vi "Controller Monitoring Loop.vi"(7 "Sync Objects":T1, 8 "error in (no error)":errorcluster, 11 "FOFB Configuration":T4={"FOFB Parameters"={"Network"={"FOFB Controller IP"="", "LNLS Control Network IP"="", "LNLS Control Network Power Supplies TCP Port"=0, "LNLS Control Network FOFB Configuration TCP Port"=0, "LNLS Control Network BPMs TCP Port"=0, "Monitoring Data TCP Port"=0, "Fast Archiver TCP Port"=0, "Fast Command TCP Port"=0, "TCP Listening Timeout"=0}, "Fast Acquisition"={"Sampling Period"=0, "Data Buffer Size"=0, "Monitoring Period"=0}, "Acquisition Network"=[], "Actuation Network"=[]}, "Number of Acquisition Chassis"=0, "Number of Actuation Chassis"=0, "Number of BPM Readings"=0, "BPM Reading Names"=[], "Selected BPM Readings"=[0, 1, 2, 3, 4, 5, 6, 7, 8, 9, 10, 11, 12, 13, 14, 15, 16, 17, 18, 19, 20, 21, 22, 23, 24, 25, 26, 27, 28, 29, 30, 31, 32, 33, 34, 35, 36, 37, 38, 39, 40, 41, 42, 43, 44, 45, 46, 47, 48, 49], "Number of Correctors"=0, "Corrector Names"=[], "Selected Correctors"=[0, 1, 2, 3, 4, 5, 6, 7, 8, 9, 10, 11, 12, 13, 14, 15, 16, 17, 18, 19, 20, 21, 22, 23, 24, 25, 26, 27, 28, 29, 30, 31, 32, 33, 34, 35, 36, 37, 38, 39, 40, 41, 42, 43, 44, 45, 46, 47, 48, 49], "Response Matrix"=[], "Reference Orbit"=[], "Correction Matrix"=[], "FPGA Filter Sets"=[], "Acquisition Chassis Names"=[], "Actuation Chassis Names"=[], "Acquisition Variables"=[], "Actuation Variables"=[], "PS Matrix Mapping"=[], "Inverse PS Matrix Mapping"=[], "BPM Matrix Mapping"=[], "Inverse BPM Matrix Mapping"=[], "BPM Planes"=[], "Corrector Planes"=[]}) -> (0 "error out":errorcluster)   [LabVIEW 2011, in "Controller VIs.lvlib"]
uses:
  Controller VIs.lvlib
  Types Definitions/Type FOFB Configuration.ctl
  Types Definitions/Type FOFB Parameters.ctl
  Types Definitions/Type Network Configuration.ctl
  Types Definitions/Type FA Configuration.ctl
  Types Definitions/Type Acquisition Network Configuration.ctl
  Types Definitions/Type Actuation Network Configuration.ctl
  Types Definitions/Type Synchronization Objects.ctl
  Types Definitions/Type Blocking Synchronization Objects.ctl
  Types Definitions/Type Monitoring Data.ctl
  Types Definitions/Type Operation Mode State.ctl
  Types Definitions/Type Diagnostics Data.ctl
  Types Definitions/Type CPU Loads Array.ctl
  Types Definitions/Type CPU Loads.ctl
  Types Definitions/Type Non-blocking Synchronization Objects.ctl
  Types Definitions/Type FOFB Variables.ctl
  Types Definitions/Type Actuation State.ctl
  Types Definitions/Type TCP State.ctl
  <vilib>/Platform/TimedLoop/XDataNode/timing_clust.ctl
  <vilib>/Platform/TimedLoop/XDataNode/nitl_modes.ctl
  <vilib>/Platform/TimedLoop/XDataNode/wakeup.ctl
  Controller Global Variables/LNLS Control FOFB Configuration Out.vi
  Controller Global Variables/Monitoring Data.vi
  <vilib>/Platform/TimedLoop/XDataNode/XDataNode.xnode
  Type Definitions.lvlib
  <vilib>/NI_Real-Time Target Support.lvlib
  Controller Global Variables.lvlib
  <vilib>/Platform/TimedLoop/XDataNode/XDNodeRunTimeDep.lvlib
  Filter VIs.lvlib
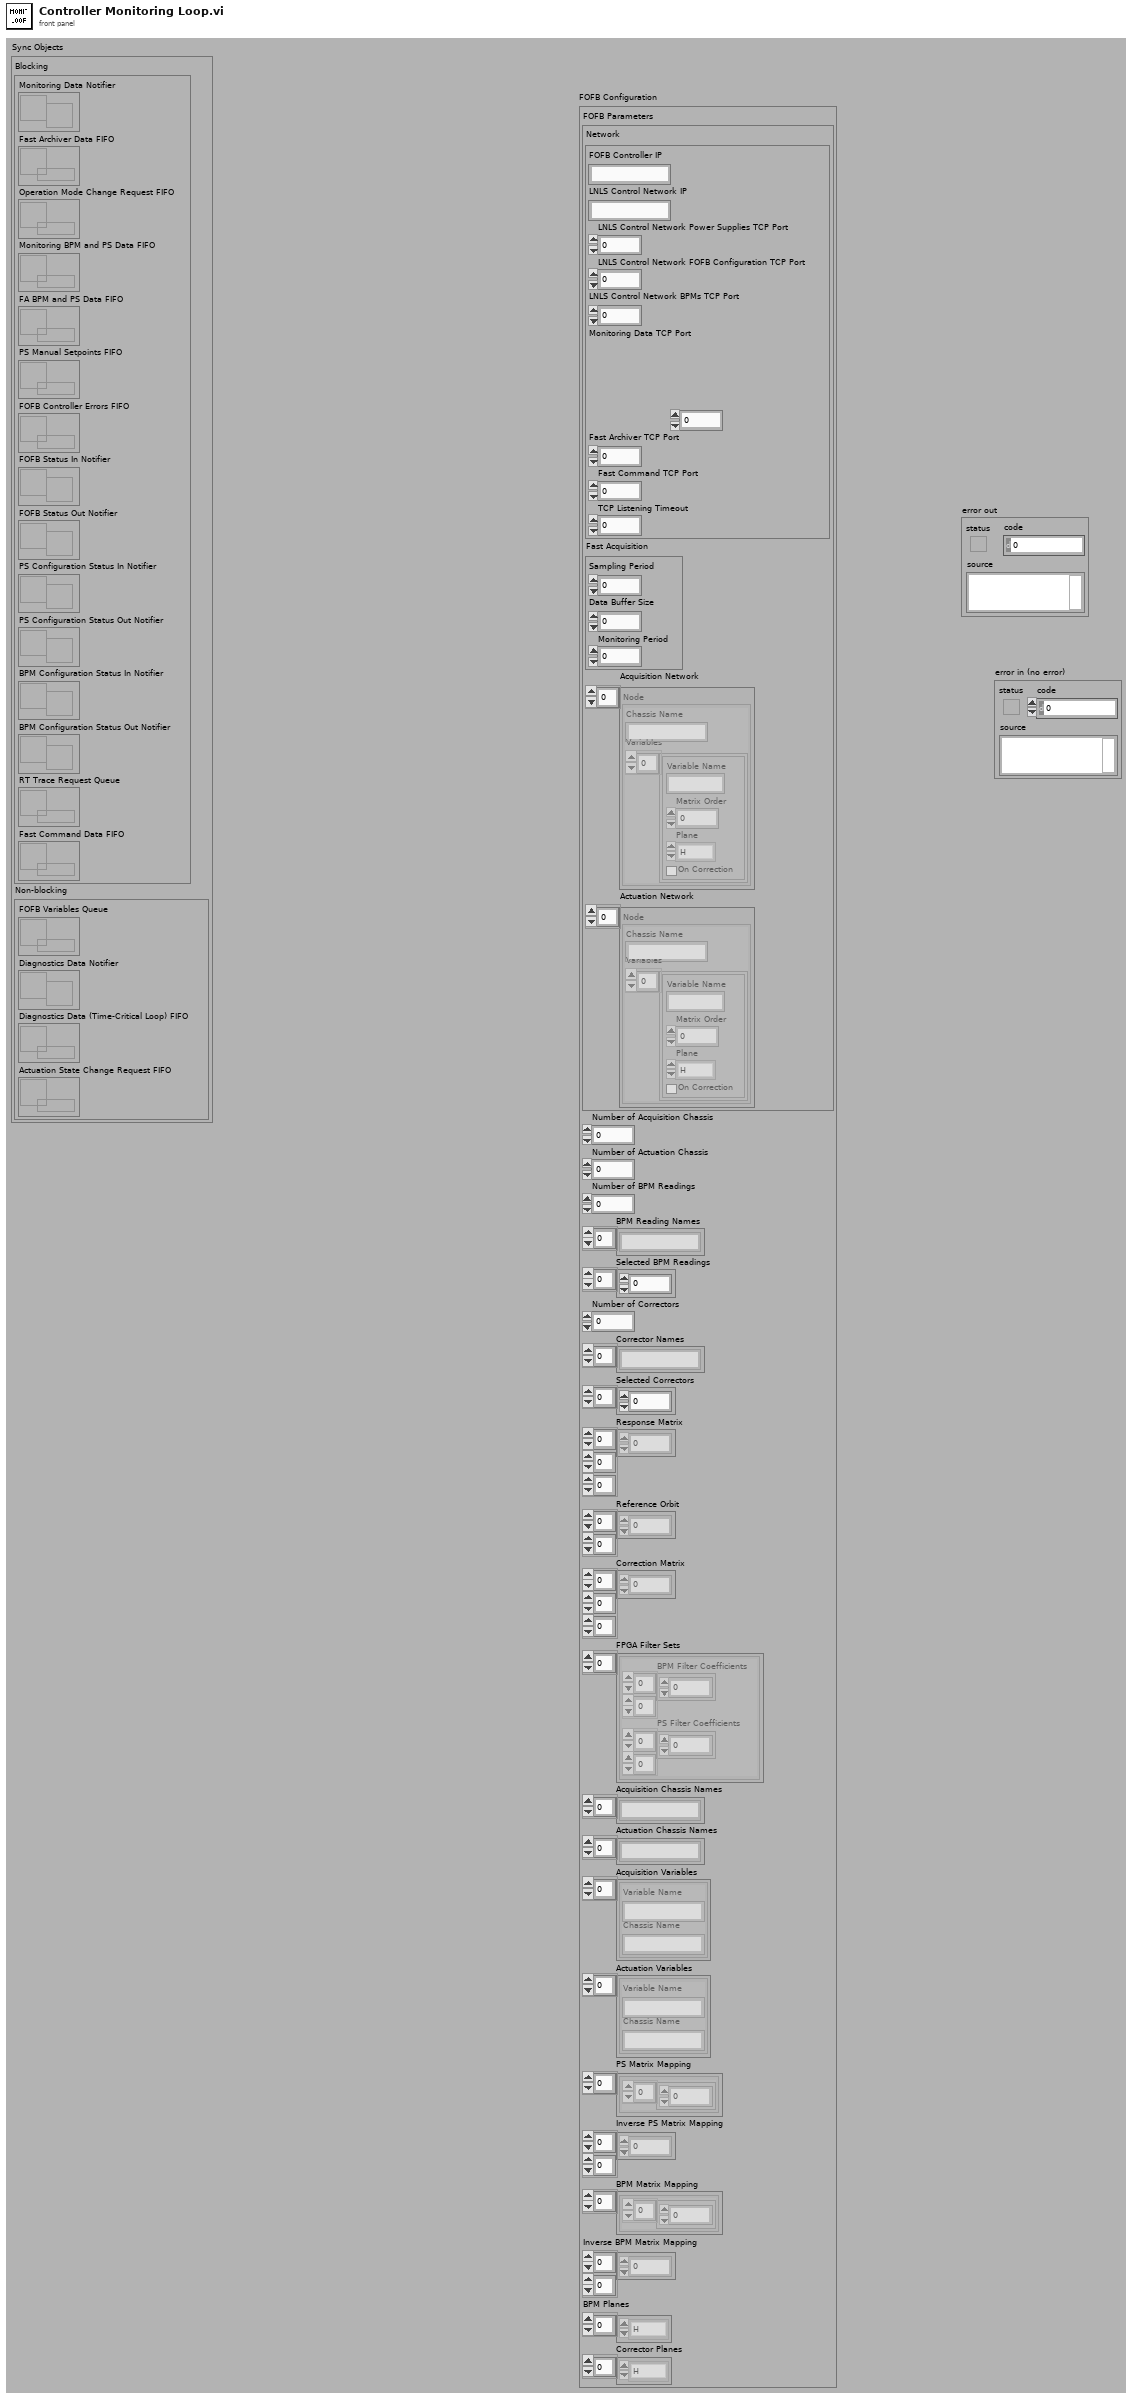
[diagram p1: front panel]
types:
  T1 = typedef "Type Definitions.lvlib/Type Synchronization Objects.ctl" = cluster{"Blocking":T2, "Non-blocking":T3}
  T2 = typedef "Type Definitions.lvlib/Type Blocking Synchronization Objects.ctl" = cluster{"Monitoring Data Notifier":refnum<notifier>, "Fast Archiver Data FIFO":refnum<queue>, "Operation Mode Change Request FIFO":refnum<k33>, "Monitoring BPM and PS Data FIFO":refnum<k33>, "FA BPM and PS Data FIFO":refnum<k33>, "PS Manual Setpoints FIFO":refnum<k33>, "FOFB Controller Errors FIFO ":refnum<k33>, "FOFB Status In Notifier":refnum<notifier>, "FOFB Status Out Notifier":refnum<notifier>, "PS Configuration Status In Notifier":refnum<notifier>, "PS Configuration Status Out Notifier":refnum<notifier>, "BPM Configuration Status In Notifier":refnum<notifier>, "BPM Configuration Status Out Notifier":refnum<notifier>, "RT Trace Request Queue":refnum<queue>, "Fast Command Data FIFO":refnum<k33>}
  T3 = typedef "Type Definitions.lvlib/Type Non-blocking Synchronization Objects.ctl" = cluster{"FOFB Variables Queue":refnum<queue>, "Diagnostics Data Notifier":refnum<notifier>, "Diagnostics Data (Time-Critical Loop) FIFO":refnum<k33>, "Actuation State Change Request FIFO":refnum<k33>}
  T4 = typedef "Type Definitions.lvlib/Type FOFB Configuration.ctl" = cluster{"FOFB Parameters":T5, "Number of Acquisition Chassis":i32, "Number of Actuation Chassis":i32, "Number of BPM Readings":i32, "BPM Reading Names":string[], "Selected BPM Readings":u32[], "Number of Correctors":i32, "Corrector Names":string[], "Selected Correctors":u32[], "Response Matrix":dbl[][][], "Reference Orbit":dbl[][], "Correction Matrix":dbl[][][], "FPGA Filter Sets":cluster{"BPM Filter Coefficients":dbl[][], "PS Filter Coefficients":dbl[][]}[], "Acquisition Chassis Names":string[], "Actuation Chassis Names":string[], "Acquisition Variables":cluster{"Variable Name":string, "Chassis Name":string}[], "Actuation Variables":cluster{"Variable Name":string, "Chassis Name":string}[], "PS Matrix Mapping":cluster{u32[]}[], "Inverse PS Matrix Mapping":u32[][], "BPM Matrix Mapping":cluster{u32[]}[], "Inverse BPM Matrix Mapping":u32[][], "BPM Planes":enum8{"H", "V"}[], "Corrector Planes":enum8{"H", "V"}[]}
  T5 = typedef "Type Definitions.lvlib/Type FOFB Parameters.ctl" = cluster{"Network":T6, "Fast Acquisition":T7, "Acquisition Network":T8, "Actuation Network":T9}
  T6 = typedef "Type Definitions.lvlib/Type Network Configuration.ctl" = cluster{"FOFB Controller IP":string, "LNLS Control Network IP":string, "LNLS Control Network Power Supplies TCP Port":u16, "LNLS Control Network FOFB Configuration TCP Port":u16, "LNLS Control Network BPMs TCP Port":u16, "Monitoring Data TCP Port":u16, "Fast Archiver TCP Port":u16, "Fast Command TCP Port":u16, "TCP Listening Timeout":i32}
  T7 = typedef "Type Definitions.lvlib/Type FA Configuration.ctl" = cluster{"Sampling Period":u32, "Data Buffer Size":u32, "Monitoring Period":u32}
  T8 = typedef "Type Definitions.lvlib/Type Acquisition Network Configuration.ctl" = cluster{"Chassis Name":string, "Variables":cluster{"Variable Name":string, "Matrix Order":u32, "Plane":enum8{"H", "V"}, "On Correction":bool}[]}[]
  T9 = typedef "Type Definitions.lvlib/Type Actuation Network Configuration.ctl" = cluster{"Chassis Name":string, "Variables":cluster{"Variable Name":string, "Matrix Order":u32, "Plane":enum8{"H", "V"}, "On Correction":bool}[]}[]
  T10 = typedef "Type Definitions.lvlib/Type TCP State.ctl" = enum16{"Idle", "Wait Connection", "Read Data", "Process Data", "Write Data", "Close Connection"}
  T11 = typedef "XDNodeRunTimeDep.lvlib/timing_clust.ctl" = cluster{"Expected End [f-1]":u64, "Actual End [f-1]":u64, "Finished Late? [f-1]":bool, "Expected End [i-1]":u64, "Actual End [i-1]":u64, "Finished Late? [i-1]":bool, "Expected Start [i]":u64, "Actual Start [i]":u64, "Expected Start [f]":u64, "Actual Start [f]":u64, "Source Name":string, "Structure Name":string, "Period":i64, "Deadline":i64, "Offset":i64, "Start":i64, "Priority":i32, "Timeout":i32, "Mode":T12, "Wakeup Reason":T13, "Error":errorcluster, "Source Type":string, "Secondary Source Type":string, "Global End Time":u64, "Global Start Time":u64, "Frame Duration":u64, "Iteration Duration":u64, "Assigned CPU":i32, "I/O Scan Engine Mode":u32}
  T12 = typedef "XDNodeRunTimeDep.lvlib/nitl_modes.ctl" = enum32{"No Change", "Process missed periods, maintain original phase", "Discard missed periods, maintain original phase", "Process missed periods, ignore original phase", "Discard missed periods, ignore original phase"}
  T13 = typedef "XDNodeRunTimeDep.lvlib/wakeup.ctl" = enum32{"Normal", "Aborted", "Asynchronous wakeup", "Timing source error", "Timed loop error", "Timeout"}
  T14 = typedef "Type Definitions.lvlib/Type Monitoring Data.ctl" = cluster{"Timestamp":timestamp, "BPM Readings":dbl[], "PS Readings":dbl[], "PS FOFB Setpoints":dbl[], "PS Status per Rack":u8[], "PS ON-OFF per Rack":u8[], "Operation Mode":T15, "Diagnostics Data":T16, "Controller Status Table":i32[]}
  T15 = typedef "Type Definitions.lvlib/Type Operation Mode State.ctl" = enum8{"Idle Mode", "Manual Mode", "FOFB Mode"}
  T16 = typedef "Type Definitions.lvlib/Type Diagnostics Data.ctl" = cluster{"Time-Critical Loop Missed Iterations":u32, "Time-Critical Loop Execution Time (usec)":u32, "Available Memory (bytes)":u32, "CPU Loads Array":T17}
  T17 = typedef "Type Definitions.lvlib/Type CPU Loads Array.ctl" = T18[]
  T18 = typedef "Type Definitions.lvlib/Type CPU Loads.ctl" = cluster{"Total (%)":dbl, "Time Critical (%)":dbl, "Timed Structures (%)":dbl, "High (%)":dbl, "Above Normal (%)":dbl, "Normal (%)":dbl, "Background (%)":dbl, "Idle (%)":dbl, "ISR (%)":dbl}
  T19 = typedef "Type Definitions.lvlib/Type Control FOFB Configuration Out.ctl" = cluster{"Status":u16, "Operation Mode":T15, "Horizontal Gain":sgl, "Vertical Gain":sgl, "Selected Reference Orbit":i32, "Selected Correction Matrix":i32, "Selected FPGA Filters":i32, "Horizontal Distortion Threshold":sgl, "Vertical Distortion Threshold":sgl, "Timestamp":dbl}
  T20 = typedef "NI_Real-Time Target Support.lvlib/RT CPU Load.ctl" = cluster{"Total (%)":dbl, "Time Critical (%)":dbl, "Timed Structures (%)":dbl, "High (%)":dbl, "Above Normal (%)":dbl, "Normal (%)":dbl, "Background (%)":dbl, "Idle (%)":dbl, "ISR (%)":dbl}
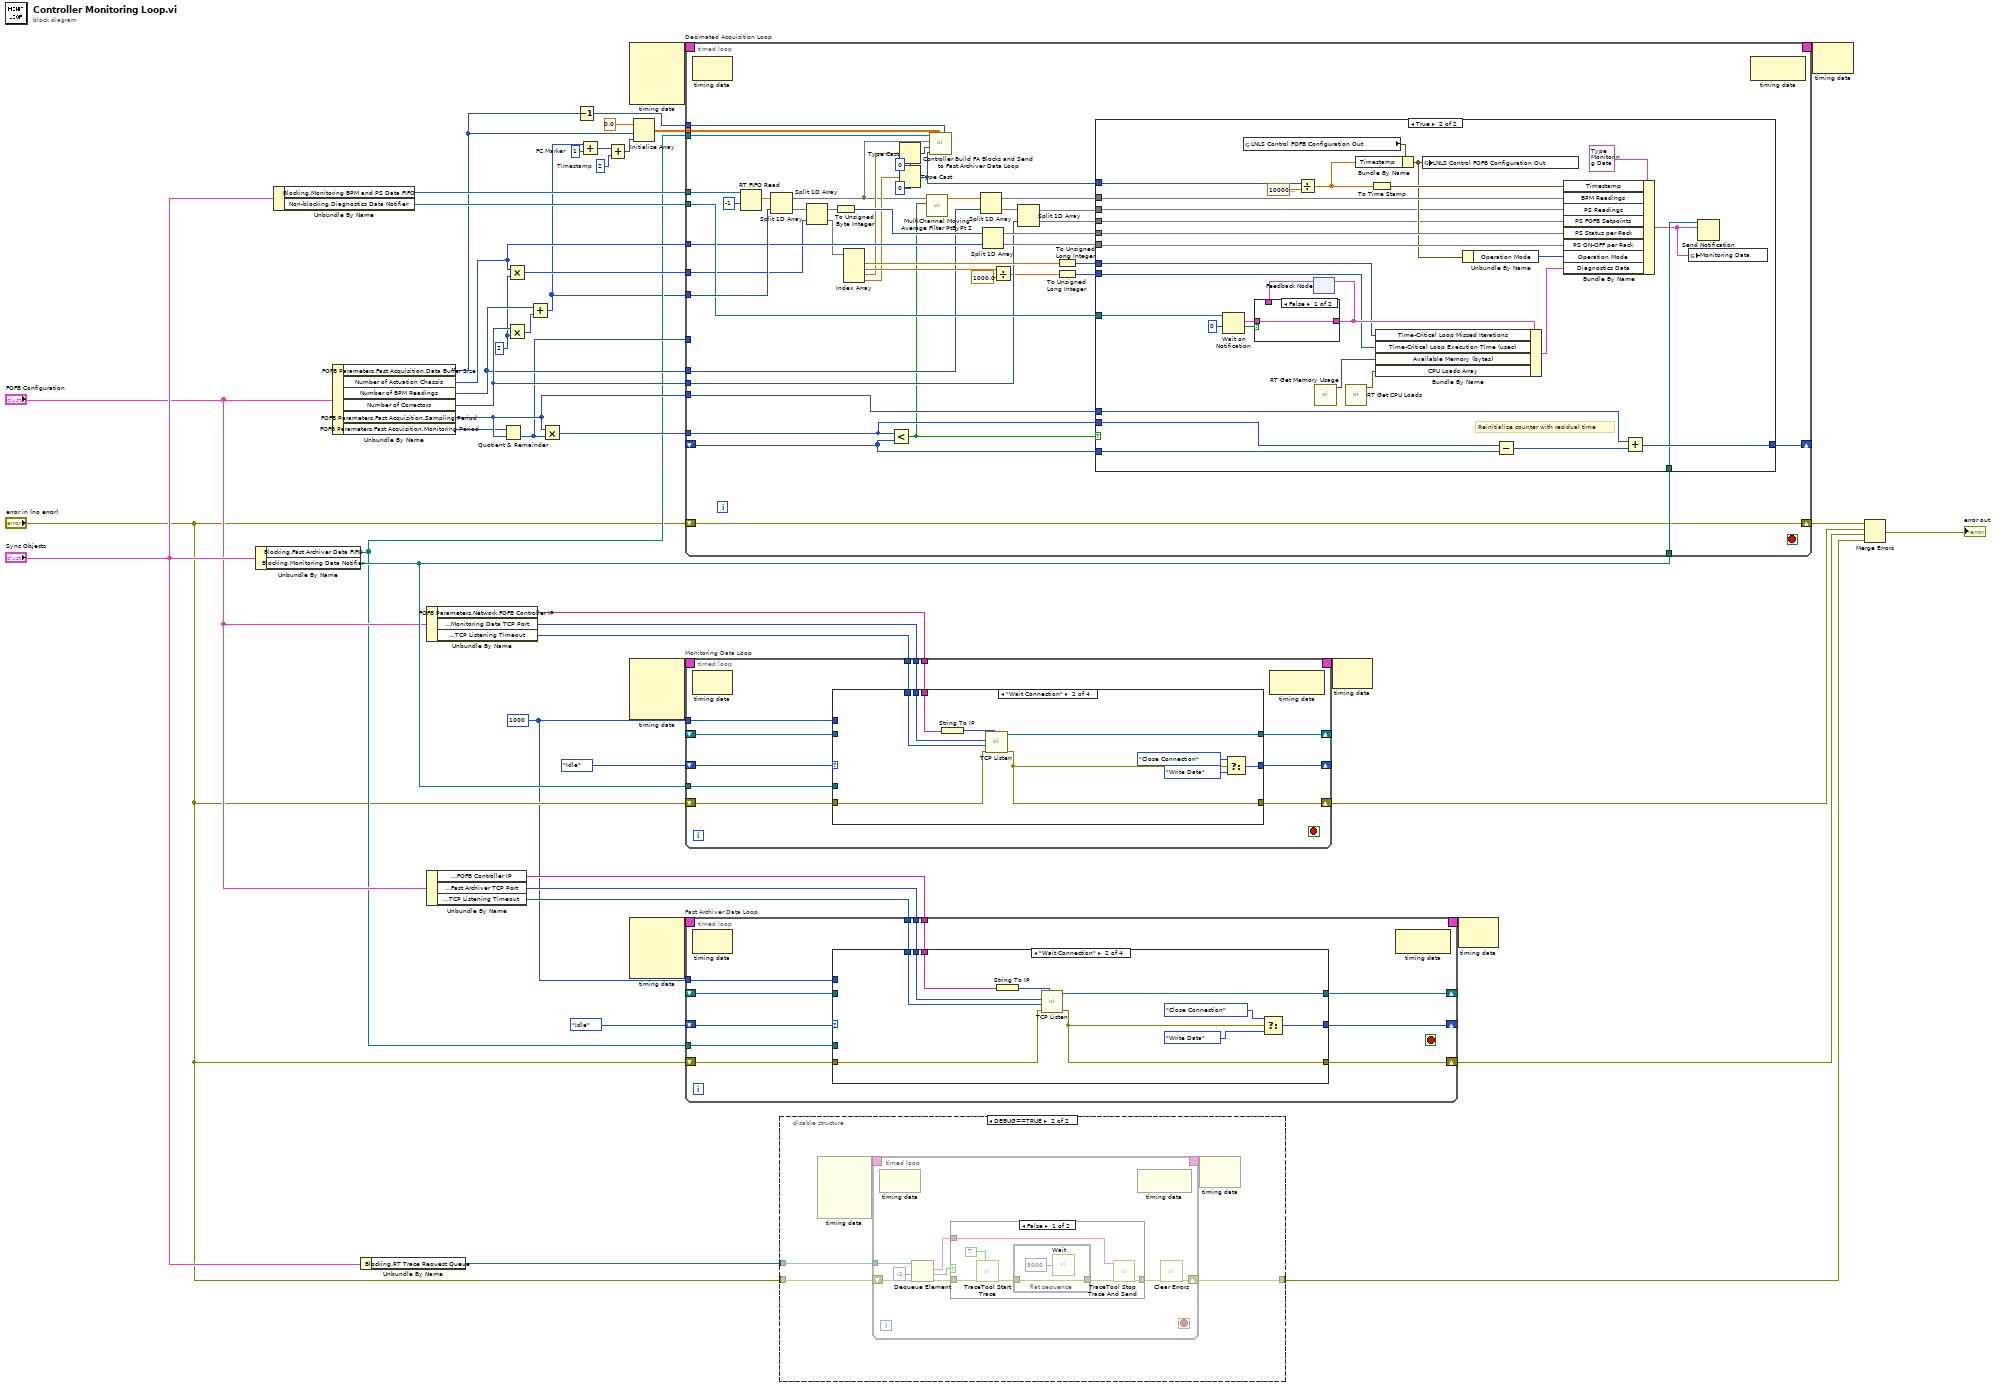
[diagram p0: block diagram]
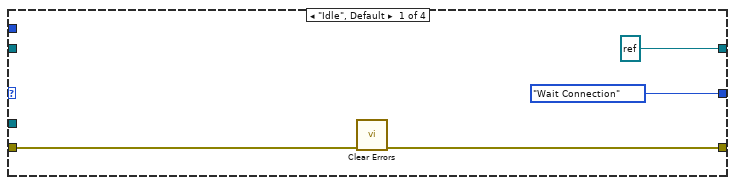
[diagram p4: hidden frame]
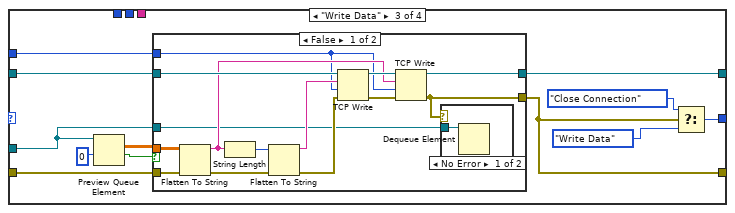
[diagram p5: hidden frame]
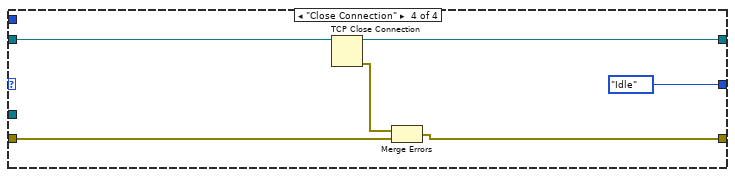
[diagram p8: hidden frame]
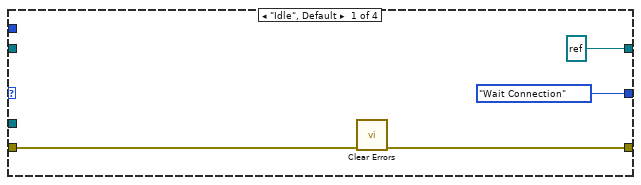
[diagram p9: hidden frame]
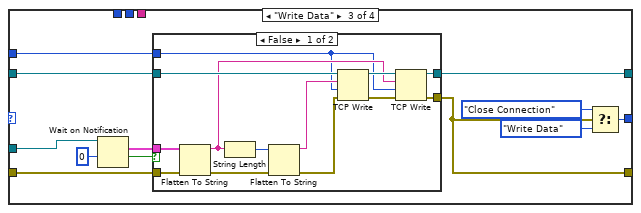
[diagram p10: hidden frame]
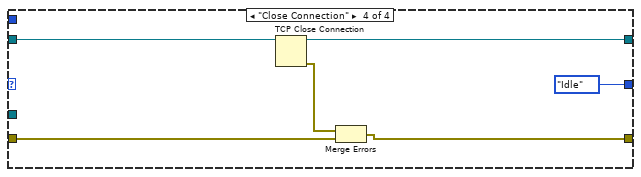
[diagram p12: hidden frame]
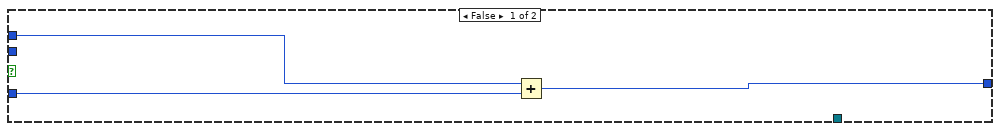
[diagram p13: hidden frame]
diagram:
  w3 = 2  # Timestamp
  w4 = 1000 ("TCP Listening Timeout")
  w8 = 1  # FC Marker
  w36 = 2 ("y")
  n1 = Unbundle By Name("Sync Objects") -> ("Blocking.Fast Archiver Data FIFO"=w14:refnum<queue>, "Blocking.Monitoring Data Notifier"=w25:refnum<notifier>)
  n2 = Unbundle By Name("Sync Objects") -> ("Blocking.Monitoring BPM and PS Data FIFO"=w15:refnum<k33>, "Non-blocking.Diagnostics Data Notifier"=w37:refnum<notifier>)
  n3 = Unbundle By Name("FOFB Configuration") -> ("FOFB Parameters.Fast Acquisition.Data Buffer Size"=w5:u32, "Number of Actuation Chassis"=w35:i32, "Number of BPM Readings"=w39:i32, "Number of Correctors"=w40:i32, "FOFB Parameters.Fast Acquisition.Sampling Period"=w33:u32, "FOFB Parameters.Fast Acquisition.Monitoring Period"=w23:u32)
  n4 = Unbundle By Name("Sync Objects") -> ("Blocking.RT Trace Request Queue"=w29:refnum<queue>)
  n5 = Unbundle By Name("FOFB Configuration") -> ("FOFB Parameters.Network.FOFB Controller IP"=w47:string, "FOFB Parameters.Network.Monitoring Data TCP Port"=w42:u16, "FOFB Parameters.Network.TCP Listening Timeout"=w46:i32)
  n6 = Unbundle By Name("FOFB Configuration") -> ("FOFB Parameters.Network.FOFB Controller IP"=w21:string, "FOFB Parameters.Network.Fast Archiver TCP Port"=w20:u16, "FOFB Parameters.Network.TCP Listening Timeout"=w19:i32)
  n7 = Quotient & Remainder(x=w23, y=w33) -> (floor(x/y)=w32:u32)  [unwired: 1 out]
  n8 = Multiply(x=w40, y=w36) -> (x*y=w38:i32)
  n9 = Multiply(x=w35, y=w36) -> (x*y=w34:i32)
  n10 = Add(x=w39, y=w38) -> (x+y=w7:i32)
  n11 = Multiply(x=w33, y=w32) -> (x*y=w24:u32)
  n12 = Decrement(x=w5) -> (x-1=w6:u32)
  n13 = Add(x=w7, y=w8) -> (x+y=w2:i32)
  n14 = Add(x=w2, y=w3) -> (x+y=w1:i32)
  n15 = node-c288() -> (w31:T11)  [unwired: 4 in]
  n16 = node-c288() -> (w27:T11)  [unwired: 4 in]
  n17 = node-c288() -> (w12:T11)  [unwired: 4 in]
  n18 = Initialize Array(sgl 0.0 ("element"), w5, w1) -> (w9:sgl[][])
  n19 = timed-loop "Decimated Acquisition Loop" {
    shift-right: [w59] -> w45
    shift-left: "error in (no error)" -> [w59]
    tunnel: w39 -> [w66]
    tunnel: w40 -> [w65]
    tunnel: w33 -> [w87]
    tunnel: w24 -> [w86]
    tunnel: w25 -> [w85]
    tunnel: w32 -> [_]
    shift-right: [w83] -> _
    shift-left: _ -> [w84]
    tunnel: w7 -> [w80]
    tunnel: w37 -> [w79]
    tunnel: w35 -> [w75]
    tunnel: w34 -> [w72]
    timing: w31 -> [_]
    timing-out: [_] -> w30
    tunnel: w9 -> [w57]
    tunnel: w6 -> [w56]
    tunnel: w15 -> [w62]
    tunnel: w14 -> [w61]
    stop <- _ stop-if-true
    n20 = node-c288() -> ()  [unwired: 1 in, 1 out]
    n21 = RT FIFO Read(0:w62, 2:-1 ("timeout in ms (0)")) -> (9:w81:dbl[])  [unwired: 2 in, 4 out]
    n22 = Split 1D Array(array=w81, index=w80) -> (first subarray=w50:dbl[], second subarray=w74:dbl[])
    n23 = Split 1D Array(array=w74, index=w72) -> (first subarray=w73:dbl[], second subarray=w60:dbl[])
    n24 = To Unsigned Byte Integer(number=w73) -> (unsigned 8bit integer=w78:u8[])
    n25 = Index Array(array=w60) -> (element #1=w70:dbl, element #2=w69:dbl, element #3=w53:dbl, element #4=w55:dbl)  [unwired: 4 in]
    n26 = Less?(x=w86, y=w84) -> (x < y?=w48:bool)
    n27 = Type Cast(type=u32 0 ("n"), x=w53) -> (*(type *) &x=w51:u32)
    n28 = Type Cast(type=u64 0 ("n"), x=w55) -> (*(type *) &x=w52:u64)
    n29 = call "MultiChannel Moving Average Filter PtByPt 2.vi"("sample?"=w48, "x"=w50) -> ("Array"=w49:dbl[])  [unwired: 9 in]
    n30 = call "Controller Build FA Blocks and Send to Fast Archiver Data Loop.vi"("Number of Blocks"=w56, "FA Data (Zeroed)"=w57, "Timestamp"=w52, "FC Marker"=w51, "FA Data (BPM Readings / PS Readings / PS Setpoints)"=w50, "Queue in"=w61) -> ()  [unwired: 6 in]
    n31 = Split 1D Array(array=w49, index=w66) -> (first subarray=w67:dbl[], second subarray=w90:dbl[])
    n32 = Split 1D Array(array=w78, index=w75) -> (first subarray=w77:u8[], second subarray=w76:u8[])
    n33 = Divide(x=w69, y=1000.0) -> (x/y=w64:dbl)
    n34 = Split 1D Array(array=w90, index=w65) -> (first subarray=w89:dbl[], second subarray=w88:dbl[])
    n35 = To Unsigned Long Integer(number=w70) -> (unsigned 32bit integer=w71:u32)
    n36 = To Unsigned Long Integer(number=w64) -> (unsigned 32bit integer=w63:u32)
    n37 = case shown="True" w48 {
      tunnel: w67 -> [_ w121]
      tunnel: w89 -> [_ w97]
      tunnel: w88 -> [_ w96]
      tunnel: [w93 w125] -> w83
      tunnel: w84 -> [w94 w124]
      tunnel: w86 -> [_ w123]
      tunnel: w87 -> [w95 w122]
      tunnel: w85 -> [_ w105]
      tunnel: w77 -> [_ w117]
      tunnel: w79 -> [_ w111]
      tunnel: w76 -> [_ w110]
      tunnel: w71 -> [_ w107]
      tunnel: w63 -> [_ w108]
      tunnel: w52 -> [_ w102]
      frame False {
        n38 = Add(x=w95, y=w94) -> (x+y=w93:u32)
      }
      frame True {
        # "Reinitialize counter with residual time"
        n39 = Wait on Notification(notifier=w111, timeout in ms (-1)=0) -> (notification=w113:T16, timed out?=w114:bool)  [unwired: 2 in, 2 out]
        n40 = global read "LNLS Control FOFB Configuration Out.vi" "LNLS Control FOFB Configuration Out"() -> (w101:T19)
        n41 = Divide(x=w102, y=1000000000.0) -> (x/y=w99:dbl)
        n42 = feedback #1() -> (w115:T16)  [unwired: 1 in]
        n43 = case shown="False" w114 {
          tunnel: [w127 w128] -> w112
          tunnel: w113 -> [w127 _]
          tunnel: w115 -> [_ w128]
          frame False {
          }
          frame True {
          }
        }
        n44 = feedback-in #1(w112) -> ()
        n45 = call <vilib>:"RT Get Memory Usage.vi"() -> ("total (bytes)"=w109:u32)  [unwired: 8 in, 3 out]
        n46 = call <vilib>:"RT Get CPU Loads.vi"() -> ("CPU loads"=w119:T20[])  [unwired: 10 in, 1 out]
        n47 = Bundle By Name(cluster=w101, "Timestamp"=w99) -> (w98:T19)
        n48 = To Time Stamp(1:w99) -> (0:w100:timestamp)
        n49 = Bundle By Name(cluster=w112, "Time-Critical Loop Missed Iterations"=w107, "Time-Critical Loop Execution Time (usec)"=w108, "Available Memory (bytes)"=w109, "CPU Loads Array"=w119) -> (w118:T16)
        n50 = global write "LNLS Control FOFB Configuration Out.vi" "LNLS Control FOFB Configuration Out"(w98) -> ()
        n51 = Unbundle By Name(w98) -> ("Operation Mode"=w106:T15)
        n52 = Subtract(x=w123, y=w124) -> (x-y=w126:u32)
        n53 = Bundle By Name(cluster=T14 {"Timestamp"=timestamp(0 s since 1904-01-01), "BPM Readings"=[], "PS Readings"=[], "PS FOFB Setpoints"=[], "PS Status per Rack"=[], "PS ON-OFF per Rack"=[], "Operation Mode"=enum."Idle Mode", "Diagnostics Data"={"Time-Critical Loop Missed Iterations"=0, "Time-Critical Loop Execution Time (usec)"=0, "Available Memory (bytes)"=0, "CPU Loads Array"=[]}, "Controller Status Table"=[]} ("output cluster"), "Timestamp"=w100, "BPM Readings"=w121, "PS Readings"=w97, "PS FOFB Setpoints"=w96, "PS Status per Rack"=w117, "PS ON-OFF per Rack"=w110, "Operation Mode"=w106, "Diagnostics Data"=w118) -> (w104:T14)
        n54 = Add(x=w122, y=w126) -> (x+y=w125:u32)
        n55 = global write "Monitoring Data.vi" "Monitoring Data"(w104) -> ()
        n56 = Send Notification(notification=w104, notifier=w105) -> ()  [unwired: 1 in, 2 out]
      }
    }
    n57 = node-c288() -> ()  [unwired: 1 in, 1 out]
  }
  n58 = timed-loop "Monitoring Data Loop" {
    tunnel: w47 -> [w139]
    tunnel: w42 -> [w138]
    tunnel: w46 -> [w137]
    shift-right: [w129] -> w44
    shift-left: "error in (no error)" -> [w132]
    tunnel: w25 -> [w131]
    shift-right: [w135] -> _
    shift-left: Type_TCP_State."Idle" ("f") -> [w136]
    shift-right: [w133] -> _
    shift-left: _ -> [w134]
    timing: w27 -> [_]
    timing-out: [_] -> w26
    tunnel: w4 -> [w130]
    stop <- _ stop-if-true
    n59 = node-c288() -> ()  [unwired: 1 in, 1 out]
    n60 = case shown="\"Wait Connection\"" w136 {
      tunnel: [refnum<k5> refnum ("connection ID") w155 w167 w188] -> w133
      tunnel: [Type_TCP_State."Wait Connection" ("f") w154 w166 Type_TCP_State."Idle" ("f")] -> w135
      tunnel: [w142 w150 w162 w183] -> w129
      tunnel: w132 -> [w143 w151 w158 w184]
      tunnel: w134 -> [_ _ w163 w186]
      tunnel: w139 -> [_ w147 _ _]
      tunnel: w138 -> [_ w149 _ _]
      tunnel: w137 -> [_ w146 _ _]
      tunnel: w131 -> [_ _ w161 _]
      tunnel: w130 -> [_ _ w156 _]
      frame "Idle", Default {
        n61 = call <vilib>:"Clear Errors.vi"("error in (no error)"=w143) -> ("error out"=w142:errorcluster)  [unwired: 6 in]
      }
      frame "Wait Connection" {
        n62 = String To IP(1:w147) -> (0:w148:u32)
        n63 = call <vilib>:"TCP Listen.vi"("net address"=w148, "error in (no error)"=w151, "timeout ms (wait forever: -1)"=w146, "port"=w149) -> ("error out"=w150:errorcluster, "connection ID"=w155:refnum<k5>)  [unwired: 3 in, 3 out]
        n64 = Select(t=Type_TCP_State."Close Connection" ("f"), s=w150, f=Type_TCP_State."Write Data") -> (s? t:f=w154:T10)
      }
      frame "Write Data" {
        n65 = Wait on Notification(notifier=w161, timeout in ms (-1)=0) -> (notification=w160:T14, timed out?=w157:bool)  [unwired: 2 in, 2 out]
        n66 = case shown="False" w157 {
          tunnel: [w180 w182] -> w167
          tunnel: w163 -> [w178 w182]
          tunnel: w156 -> [w171 _]
          tunnel: [w170 w181] -> w162
          tunnel: w160 -> [w169 _]
          tunnel: w158 -> [w168 w181]
          frame False {
            n67 = Flatten To String(anything=w169, error in (no error)=w168) -> (data string=w174:string, error out=w173:errorcluster)  [unwired: 2 in, 1 out]
            n68 = String Length(string=w174) -> (length=w176:i32)
            n69 = Flatten To String(anything=w176, error in (no error)=w173) -> (data string=w175:string, error out=w172:errorcluster)  [unwired: 2 in, 1 out]
            n70 = TCP Write(connection ID=w178, data in=w175, error in (no error)=w172, 9:w171) -> (connection ID out=w179:refnum<k5>, error out=w177:errorcluster)  [unwired: 1 out]
            n71 = TCP Write(connection ID=w179, data in=w174, error in (no error)=w177, 9:w171) -> (connection ID out=w180:refnum<k5>, error out=w170:errorcluster)  [unwired: 1 out]
          }
          frame True {
          }
        }
        n72 = Select(t=Type_TCP_State."Close Connection" ("f"), s=w162, f=Type_TCP_State."Write Data") -> (s? t:f=w166:T10)
      }
      frame "Close Connection" {
        n73 = TCP Close Connection(connection ID=w186) -> (connection ID out=w188:refnum<k5>, error out=w185:errorcluster)  [unwired: 2 in]
        n74 = Merge Errors(w185, w184) -> (w183:errorcluster)
      }
    }
    n75 = node-c288() -> ()  [unwired: 1 in, 1 out]
  }
  n76 = timed-loop "Fast Archiver Data Loop" {
    tunnel: w21 -> [w199]
    tunnel: w20 -> [w198]
    tunnel: w19 -> [w197]
    shift-right: [w189] -> w17
    shift-left: "error in (no error)" -> [w192]
    tunnel: w14 -> [w191]
    shift-right: [w195] -> _
    shift-left: Type_TCP_State."Idle" ("f") -> [w196]
    shift-right: [w193] -> _
    shift-left: _ -> [w194]
    timing: w12 -> [_]
    timing-out: [_] -> w11
    tunnel: w4 -> [w190]
    stop <- _ stop-if-true
    n77 = node-c288() -> ()  [unwired: 1 in, 1 out]
    n78 = case shown="\"Wait Connection\"" w196 {
      tunnel: [refnum<k5> refnum ("connection ID") w215 w227 w250] -> w193
      tunnel: [Type_TCP_State."Wait Connection" ("f") w214 w226 Type_TCP_State."Idle" ("f")] -> w195
      tunnel: [w202 w210 w222 w245] -> w189
      tunnel: w192 -> [w203 w211 w221 w246]
      tunnel: w194 -> [_ _ w223 w248]
      tunnel: w199 -> [_ w207 _ _]
      tunnel: w198 -> [_ w209 _ _]
      tunnel: w197 -> [_ w206 _ _]
      tunnel: w191 -> [_ _ w219 _]
      tunnel: w190 -> [_ _ w216 _]
      frame "Idle", Default {
        n79 = call <vilib>:"Clear Errors.vi"("error in (no error)"=w203) -> ("error out"=w202:errorcluster)  [unwired: 6 in]
      }
      frame "Wait Connection" {
        n80 = String To IP(1:w207) -> (0:w208:u32)
        n81 = call <vilib>:"TCP Listen.vi"("net address"=w208, "error in (no error)"=w211, "timeout ms (wait forever: -1)"=w206, "port"=w209) -> ("error out"=w210:errorcluster, "connection ID"=w215:refnum<k5>)  [unwired: 3 in, 3 out]
        n82 = Select(t=Type_TCP_State."Close Connection" ("f"), s=w210, f=Type_TCP_State."Write Data") -> (s? t:f=w214:T10)
      }
      frame "Write Data" {
        n83 = Preview Queue Element(queue=w219, timeout in ms (-1)=0) -> (element=w218:sgl[][], timed out?=w220:bool)  [unwired: 1 in, 2 out]
        n84 = case shown="False" w220 {
          tunnel: [w241 w244] -> w227
          tunnel: w223 -> [w239 w244]
          tunnel: w216 -> [w232 _]
          tunnel: [w229 w243] -> w222
          tunnel: w218 -> [w231 _]
          tunnel: w221 -> [w230 w243]
          tunnel: w219 -> [w228 _]
          frame False {
            n85 = Flatten To String(anything=w231, error in (no error)=w230) -> (data string=w235:string, error out=w234:errorcluster)  [unwired: 2 in, 1 out]
            n86 = String Length(string=w235) -> (length=w237:i32)
            n87 = Flatten To String(anything=w237, error in (no error)=w234) -> (data string=w236:string, error out=w233:errorcluster)  [unwired: 2 in, 1 out]
            n88 = TCP Write(connection ID=w239, data in=w236, error in (no error)=w233, 9:w232) -> (connection ID out=w240:refnum<k5>, error out=w238:errorcluster)  [unwired: 1 out]
            n89 = TCP Write(connection ID=w240, data in=w235, error in (no error)=w238, 9:w232) -> (connection ID out=w241:refnum<k5>, error out=w229:errorcluster)  [unwired: 1 out]
            n90 = case shown="No Error" w229 {
              tunnel: w228 -> [w242 _]
              frame No Error {
                n91 = Dequeue Element(queue=w242) -> ()  [unwired: 2 in, 4 out]
              }
              frame Error {
              }
            }
          }
          frame True {
          }
        }
        n92 = Select(t=Type_TCP_State."Close Connection" ("f"), s=w222, f=Type_TCP_State."Write Data") -> (s? t:f=w226:T10)
      }
      frame "Close Connection" {
        n93 = TCP Close Connection(connection ID=w248) -> (connection ID out=w250:refnum<k5>, error out=w247:errorcluster)  [unwired: 2 in]
        n94 = Merge Errors(w247, w246) -> (w245:errorcluster)
      }
    }
    n95 = node-c288() -> ()  [unwired: 1 in, 1 out]
  }
  n96 = disable-structure shown="DEBUG==TRUE" {
    disable-tunnel: w29 -> [_ w253]
    disable-tunnel: [_ w252] -> w18
    disable-tunnel: "error in (no error)" -> [_ w251]
    frame condition #0 (active) {
    }
    frame condition #1 {
      n97 = node-c288() -> (w255:T11)  [unwired: 4 in]
      n98 = timed-loop {
        timing: w255 -> [_]
        timing-out: [_] -> w254
        tunnel: w253 -> [w261]
        shift-right: [w256] -> w252
        shift-left: w251 -> [w259]
        stop <- _ stop-if-true
        n99 = node-c288() -> ()  [unwired: 1 in, 1 out]
        n100 = Dequeue Element(queue=w261, timeout in ms (-1)=-1, error in (no error)=w259) -> (element=w260:string, timed out?=w262:bool, error out=w258:errorcluster)  [unwired: 1 out]
        n101 = case shown="False" w262 {
          tunnel: [w268 w272] -> w257
          tunnel: w260 -> [w267 _]
          tunnel: w258 -> [w266 w272]
          frame False {
            n102 = call <vilib>:"TraceTool Start Trace.vi"("Detailed Tracing? (F)"=TRUE, "error in (no error)"=w266) -> ("error out"=w269:errorcluster)  [unwired: 8 in, 1 out]
            n103 = flat-sequence {
              tunnel: w269 -> [w270]
              tunnel: [w270] -> w264
              frame #0 {
                n104 = call "Wait"("Count(mSec)"=u32 5000) -> ()  [unwired: 1 out]
              }
            }
            n105 = call <vilib>:"TraceTool Stop Trace And Send.vi"("error in (no error)"=w264, "Trace Host Network Address"=w267) -> ("error out"=w268:errorcluster)  [unwired: 9 in]
          }
          frame True {
          }
        }
        n106 = node-c288() -> ()  [unwired: 1 in, 1 out]
        n107 = call <vilib>:"Clear Errors.vi"("error in (no error)"=w257) -> ("error out"=w256:errorcluster)  [unwired: 6 in]
      }
      n108 = node-c288(w254) -> ()  [unwired: 1 out]
    }
  }
  n109 = node-c288(w26) -> ()  [unwired: 1 out]
  n110 = node-c288(w11) -> ()  [unwired: 1 out]
  n111 = node-c288(w30) -> ()  [unwired: 1 out]
  n112 = Merge Errors(w45, w44, w17, w18) -> (→"error out":errorcluster)
